vi "Send cmd and wait for keyword.vi"(6 "VISA resource name":refnum<visa-resource-name>, 8 "error in (no error)":errorcluster, 9 "Wait after":u32=750, 10 "Wait for":string, 11 "write buffer":string) -> (0 "error out":errorcluster, 2 "Response":string, 3 "timeout":bool, 4 "VISA Refnum out":refnum<visa-resource-name>)   [LabVIEW 2024]
panel:
  in  "Timeout (mSecs)":u32=3000
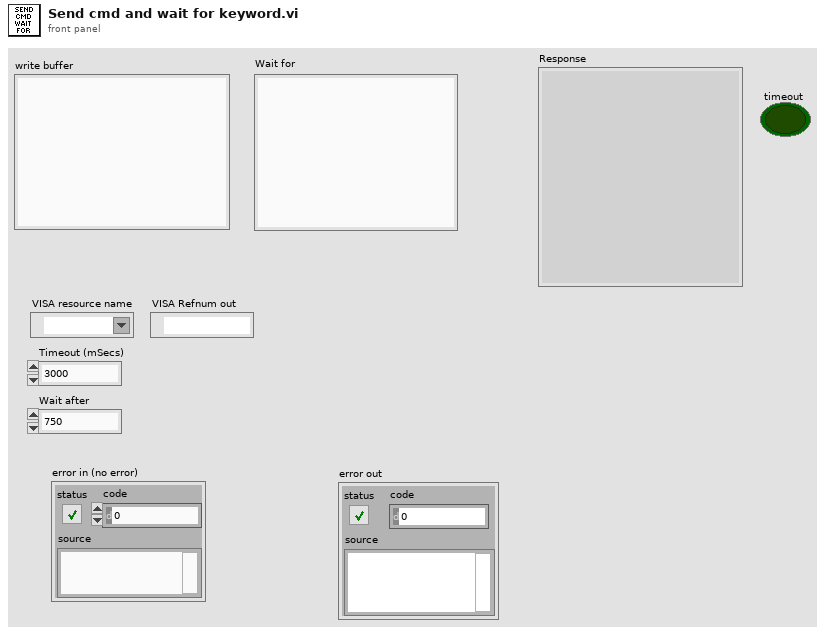
[diagram p1: front panel]
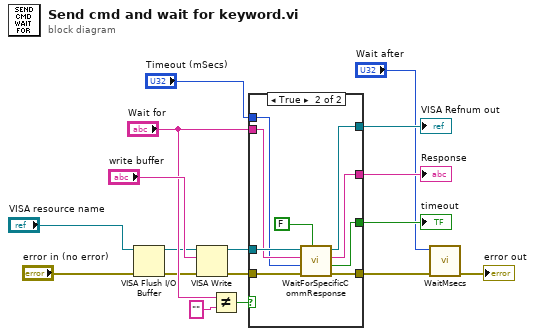
[diagram p0: block diagram]
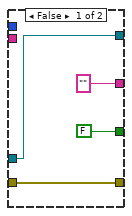
[diagram p2: hidden frame]
diagram:
  n1 = VISA Flush I/O Buffer(VISA resource name="VISA resource name", error in (no error)="error in (no error)") -> (VISA resource name out=w3:refnum<visa-resource-name>, error out=w1:errorcluster)  [unwired: 1 in]
  n2 = VISA Write(VISA resource name=w3, write buffer="write buffer", error in (no error)=w1) -> (VISA resource name out=w16:refnum<visa-resource-name>, error out=w15:errorcluster)  [unwired: 1 out]
  n3 = Not Equal?(x="Wait for", y="") -> (x != y?=w5:bool)
  n4 = case shown="True" w5 {
    tunnel: w16 -> [w21 w30]
    tunnel: w15 -> [w18 w29]
    tunnel: "Wait for" -> [_ w28]
    tunnel: "Timeout (mSecs)" -> [_ w27]
    tunnel: ["" ("Response") w25] -> w13
    tunnel: [FALSE ("timeout") w24] -> w12
    tunnel: [w21 w23] -> w11
    tunnel: [w18 w22] -> w10
    frame False {
    }
    frame True {
      n5 = call "WaitForSpecificCommResponse.vi"("Display err mess?"=FALSE, "error in (no error)"=w29, "Timeout (mSecs)"=w27, "Wait for"=w28, "VISA Refnum in"=w30) -> ("error out"=w22:errorcluster, "timeout"=w24:bool, "Response"=w25:string, "VISA Refnum out"=w23:refnum<visa-resource-name>)  [unwired: 2 in, 1 out]
    }
  }
  "VISA Refnum out" <- w11
  "Response" <- w13
  "timeout" <- w12
  n6 = call "WaitMsecs.vi"("error in (no error)"=w10, "Wait Msecs"="Wait after") -> ("error out"=→"error out":errorcluster)  [unwired: 9 in]
